vi "N2O同位素分析仪串口通讯.vi"(0 "VISA resource name":refnum<visa-resource-name>="COM3") -> (2 "温度摄氏度":string, 3 "d15NB":string, 4 "时间":string, 6 "N2O":string, 8 "d15N":string, 10 "d18O":string, 12 "超时us":string, 13 "气压Torr":string, 14 "H2O":string, 15 "d15NA":string)   [LabVIEW 2016]
uses:
  <vilib>/Instr/_visa.llb/VISA Configure Serial Port (Instr).vi
panel:
  out "结果字符串 2":string
  out "结果字符串":string
  out "返回数 2":u32
  out "read buffer":string
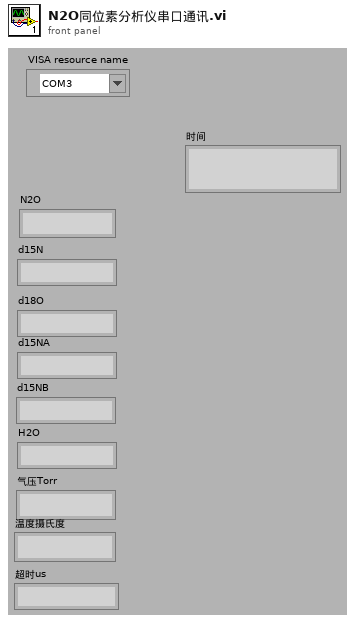
[diagram p1: front panel]
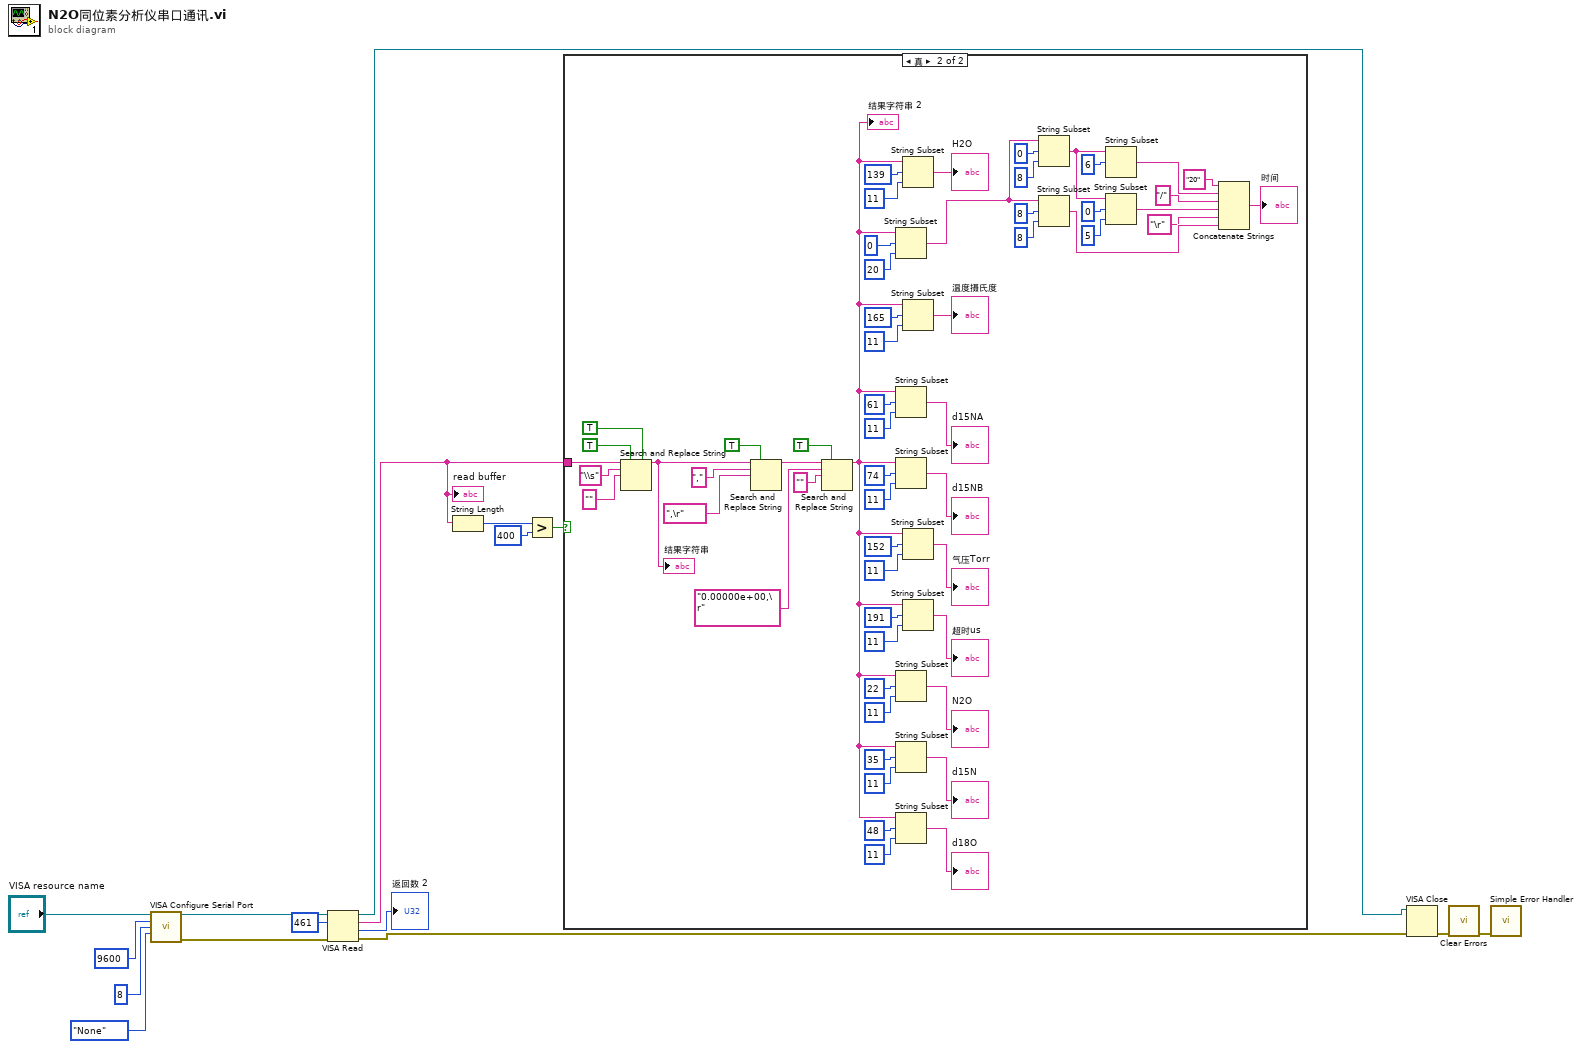
[diagram p0: block diagram]
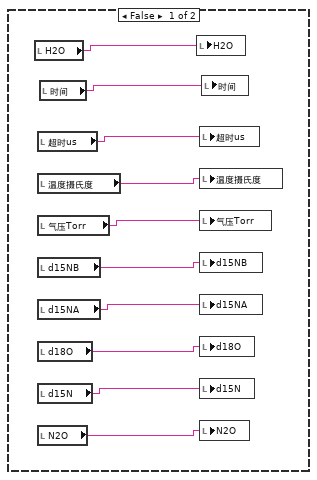
[diagram p2: hidden frame]
diagram:
  n1 = call-poly "VISA Configure Serial Port"("VISA resource name"="VISA resource name", "baud rate (9600)"=u32 9600, "data bits (8)"=u16 8, "parity (0:none)"=enum16{"None", "Odd", "Even", "Mark", "Space"}."None") -> ("VISA resource name out"=w3:refnum<visa-resource-name>, "error out"=w2:errorcluster)  [unwired: 10 in]
  n2 = VISA Read(VISA resource name=w3, byte count=u32 461 ("字节总数"), error in (no error)=w2) -> (VISA resource name out=w12:refnum<visa-resource-name>, read buffer=w4:string, return count=→"返回数 2":u32, error out=w13:errorcluster)
  "read buffer" <- w4
  n3 = String Length(string=w4) -> (length=w7:i32)
  n4 = Greater?(x=w7, y=400) -> (0:w5:bool)
  n5 = case shown="真" w5 {
    tunnel: w4 -> [_ w52]
    frame False {
      n6 = local read "H2O"() -> (w26:string)
      n7 = local read "超时us"() -> (w24:string)
      n8 = local read "温度摄氏度"() -> (w23:string)
      n9 = local read "气压Torr"() -> (w22:string)
      n10 = local read "d15NB"() -> (w21:string)
      n11 = local read "d15NA"() -> (w20:string)
      n12 = local read "d18O"() -> (w19:string)
      n13 = local read "d15N"() -> (w18:string)
      n14 = local read "N2O"() -> (w17:string)
      n15 = local read "时间"() -> (w25:string)
      n16 = local write "H2O"(w26) -> ()
      n17 = local write "超时us"(w24) -> ()
      n18 = local write "温度摄氏度"(w23) -> ()
      n19 = local write "气压Torr"(w22) -> ()
      n20 = local write "d15NB"(w21) -> ()
      n21 = local write "d15NA"(w20) -> ()
      n22 = local write "d18O"(w19) -> ()
      n23 = local write "d15N"(w18) -> ()
      n24 = local write "N2O"(w17) -> ()
      n25 = local write "时间"(w25) -> ()
    }
    frame True {
      n26 = Search and Replace String(replace all?=TRUE ("替换全部？(F)"), multiline?=TRUE ("多行？<B><B>(F)</B></B>"), input string=w52, search string="\\s" ("搜索字符串"), replace string="" ("替换字符串(\"\")")) -> (result string=w82:string)  [unwired: 3 in, 3 out]
      "结果字符串" <- w82
      n27 = Search and Replace String(replace all?=TRUE ("替换全部？(F)"), input string=w82, search string="," ("搜索字符串"), replace string=",\r" ("替换字符串(\"\")")) -> (result string=w78:string)  [unwired: 4 in, 3 out]
      n28 = Search and Replace String(replace all?=TRUE ("替换全部？(F)"), input string=w78, search string="0.00000e+00,\r" ("搜索字符串"), replace string="" ("替换字符串(\"\")")) -> (result string=w60:string)  [unwired: 4 in, 3 out]
      "结果字符串 2" <- w60
      n29 = String Subset(string=w60, offset (0)=0 ("偏移量(0)"), length (rest)=20 ("长度（剩余）")) -> (substring=w40:string)
      n30 = String Subset(string=w60, offset (0)=61 ("偏移量(0)"), length (rest)=11 ("长度（剩余）")) -> (substring=→"d15NA":string)
      n31 = String Subset(string=w60, offset (0)=74 ("偏移量(0)"), length (rest)=11 ("长度（剩余）")) -> (substring=→"d15NB":string)
      n32 = String Subset(string=w60, offset (0)=22 ("偏移量(0)"), length (rest)=11 ("长度（剩余）")) -> (substring=→"N2O":string)
      n33 = String Subset(string=w60, offset (0)=35 ("偏移量(0)"), length (rest)=11 ("长度（剩余）")) -> (substring=→"d15N":string)
      n34 = String Subset(string=w60, offset (0)=48 ("偏移量(0)"), length (rest)=11 ("长度（剩余）")) -> (substring=→"d18O":string)
      n35 = String Subset(string=w60, offset (0)=139 ("偏移量(0)"), length (rest)=11 ("长度（剩余）")) -> (substring=→"H2O":string)
      n36 = String Subset(string=w60, offset (0)=165 ("偏移量(0)"), length (rest)=11 ("长度（剩余）")) -> (substring=→"温度摄氏度":string)
      n37 = String Subset(string=w60, offset (0)=152 ("偏移量(0)"), length (rest)=11 ("长度（剩余）")) -> (substring=→"气压Torr":string)
      n38 = String Subset(string=w60, offset (0)=191 ("偏移量(0)"), length (rest)=11 ("长度（剩余）")) -> (substring=→"超时us":string)
      n39 = String Subset(string=w40, offset (0)=0 ("偏移量(0)"), length (rest)=8 ("长度（剩余）")) -> (substring=w33:string)
      n40 = String Subset(string=w40, offset (0)=8 ("偏移量(0)"), length (rest)=8 ("长度（剩余）")) -> (substring=w28:string)
      n41 = String Subset(string=w33, offset (0)=6 ("偏移量(0)")) -> (substring=w36:string)  [unwired: 1 in]
      n42 = String Subset(string=w33, offset (0)=0 ("偏移量(0)"), length (rest)=5 ("长度（剩余）")) -> (substring=w32:string)
      n43 = Concatenate Strings("20" ("字符串"), w36, "/" ("字符串"), w32, "\r" ("字符串"), w28) -> (→"时间":string)
    }
  }
  n44 = VISA Close(VISA resource name=w12, error in (no error)=w13) -> (error out=w10:errorcluster)
  n45 = call <vilib>:"Clear Errors.vi"("error in (no error)"=w10) -> ("error out"=w9:errorcluster)  [unwired: 5 in, 1 out]
  n46 = call <vilib>:"Simple Error Handler.vi"("error in (no error)"=w9) -> ()  [unwired: 4 in, 5 out]
